vi "Main_11B_X2.vi"() -> ()   [LabVIEW 2024]
uses:
  Utility/Universal Utility/TypeDefs_Utility/Cluster_Row-Column.ctl
panel:
  out "Numeric 2":i32
  out "Numeric":i32
  out "number 3":u64[](array[numeric])
  out "Count down 3":i32
  out "number 2":u64[](array[numeric])
  out "Count down 2":i32
  out "Count down":i32
  out "number":u64[](array[numeric])
  in  "Example 2":string="125 17"
  in  "Use Puzzle":bool
  out "Answer 239 for 9":u32
  in  "Puzzle":string="30 71441 3784 580926 2 8122942 0 291"
  in  "Example":string="0 1 10 99 999"
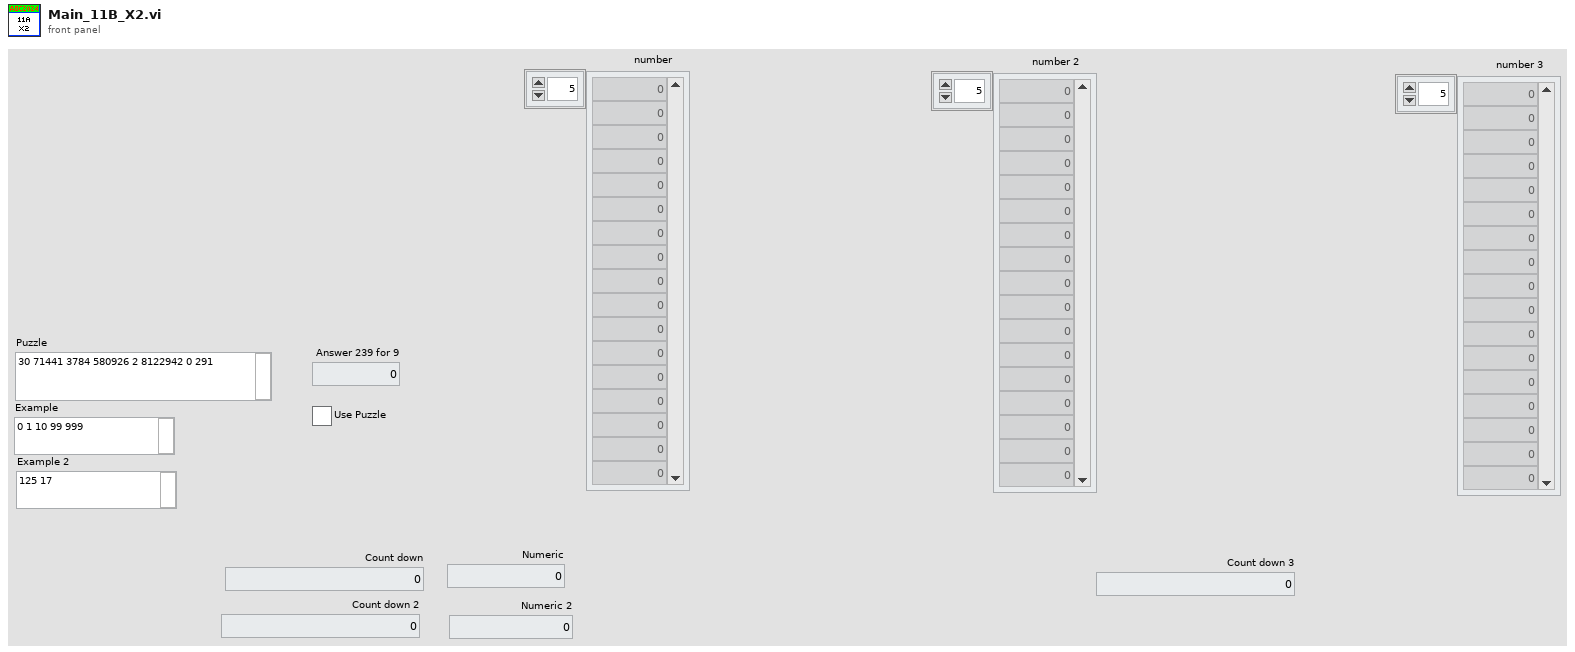
[diagram p1: front panel]
types:
  T1 = typedef "Cluster_Row-Column.ctl" = cluster{"R":i32, "C":i32}
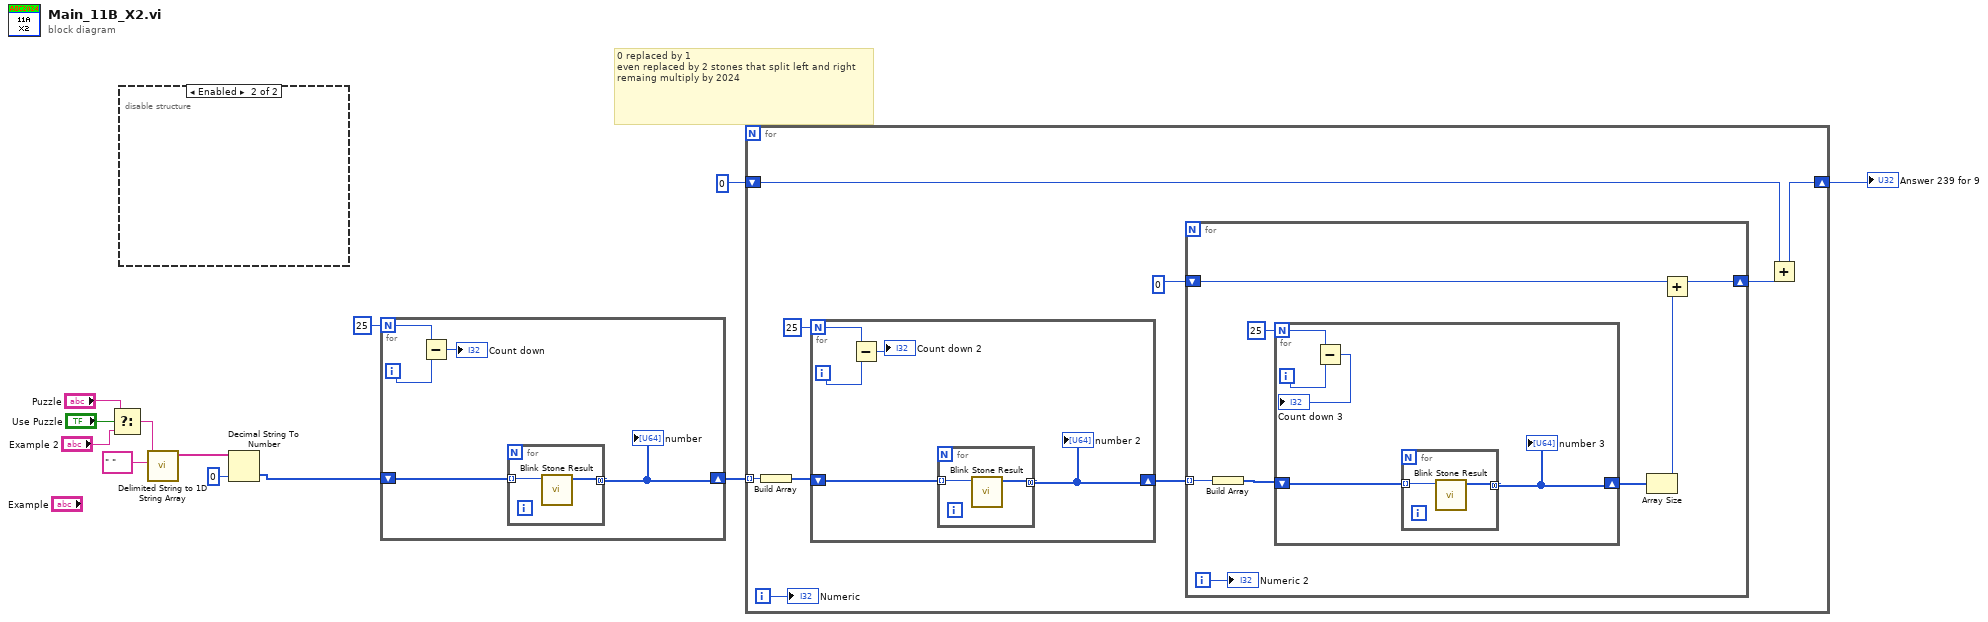
[diagram p0: block diagram]
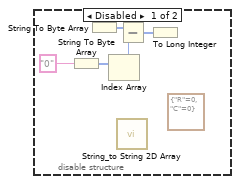
[diagram p2: hidden frame]
diagram:
  # "0 replaced by 1\neven replaced by 2 stones that split left and right\nremaing multiply by 2024"
  n1 = Select(t="Puzzle", s="Use Puzzle", f="Example 2") -> (s? t:f=w10:string)
  n2 = disable-structure shown="Enabled" {
    frame Disabled {
      (unwired) T1 {"R"=0, "C"=0} ("Position")
      n3 = String To Byte Array(string="0") -> (unsigned byte array=w17:u8[])
      n4 = String To Byte Array() -> (string=w15:string, unsigned byte array=w14:u8[])
      n5 = Index Array(array=w17) -> (element=w16:u8)  [unwired: 1 in]
      n6 = call "String_to String 2D Array.vi"() -> ()  [unwired: 11 in, 1 out]
      n7 = Subtract(x=w14, y=w16) -> (x-y=w13:u8[])
      n8 = To Long Integer(number=w13) -> ()  [unwired: 1 out]
    }
    frame Enabled {
    }
  }
  n9 = call <vilib>:"Delimited String to 1D String Array.vi"("delimiter"=" " ("delimiter (Tab)"), "delimited string"=w10) -> ("string array"=w11:string[])  [unwired: 9 in]
  n10 = Decimal String To Number(string=w11, default (0L)=u64 0 ("default (0 I32)")) -> (number=w4:u64[])  [unwired: 1 in, 1 out]
  n11 = for {
    N: 25 -> [w23]
    shift-right: [w20] -> w3
    shift-left: w4 -> [w19]
    i -> [w22]
    n12 = Subtract(x=w23, y=w22) -> (x-y=→"Count down":i32)
    n13 = for {
      tunnel: w19 -> [w25] mode=indexing
      tunnel: [w24] -> w20 mode=concatenating
      n14 = call "Blink Stone Result.vi"("String"=w25) -> ("Result Array"=w24:u64[])  [unwired: 9 in, 1 out]
    }
    "number" <- w20
  }
  n15 = for {
    tunnel: w3 -> [w33] mode=indexing
    shift-right: [w27] -> w1
    shift-left: 0 ("size(s)") -> [w28]
    i -> [w26]
    n16 = Build Array(w33) -> (w32:u64[])
    n17 = for {
      N: 25 -> [w54]
      shift-right: [w51] -> w31
      shift-left: w32 -> [w50]
      i -> [w53]
      n18 = Subtract(x=w54, y=w53) -> (x-y=→"Count down 2":i32)
      n19 = for {
        tunnel: w50 -> [w56] mode=indexing
        tunnel: [w55] -> w51 mode=concatenating
        n20 = call "Blink Stone Result.vi"("String"=w56) -> ("Result Array"=w55:u64[])  [unwired: 9 in, 1 out]
      }
      "number 2" <- w51
    }
    n21 = for {
      tunnel: w31 -> [w42] mode=indexing
      shift-right: [w36] -> w29
      shift-left: 0 ("size(s)") -> [w37]
      i -> [w35]
      n22 = Build Array(w42) -> (w41:u64[])
      n23 = for {
        N: 25 -> [w47]
        shift-right: [w44] -> w39
        shift-left: w41 -> [w43]
        i -> [w46]
        n24 = Subtract(x=w47, y=w46) -> (x-y=→"Count down 3":i32)
        n25 = for {
          tunnel: w43 -> [w49] mode=indexing
          tunnel: [w48] -> w44 mode=concatenating
          n26 = call "Blink Stone Result.vi"("String"=w49) -> ("Result Array"=w48:u64[])  [unwired: 9 in, 1 out]
        }
        "number 3" <- w44
      }
      n27 = Array Size(array=w39) -> (size(s)=w38:i32)
      n28 = Add(x=w37, y=w38) -> (x+y=w36:i32)
      "Numeric 2" <- w35
    }
    n29 = Add(x=w28, y=w29) -> (x+y=w27:i32)
    "Numeric" <- w26
  }
  "Answer 239 for 9" <- w1
